vi "CALC_EQU_VAL.vi"(0 "VISA IN":refnum<visa-resource-name>, 5 "error in":errorcluster, 7 "Channel":i32) -> (14 "VISA Out":refnum<visa-resource-name>, 18 "EqValid?":bool, 19 "error out":errorcluster)   [LabVIEW 2018, in "PNA-X.lvlib"]
doc: "CALCulate<cnum>:EQUation:VALid? \n1504\n\n(Read-Write) Returns a boolean value to indicate if the current equation on the selected measurement \nfor the specified channel is valid. For equation processing to occur, the equation must be valid and \nON (CALC:EQU:STAT 1). \nSee Critical Note \nParameters \n<cnum> Channel number of the measurement. There must be a selected measurement \non that channel. If unspecified, <cnum> is set to 1. \nExamples CALC:EQU:VAL? \ncalculate2:equation:valid? \nReturn Type Boolean \n1 - equation is valid \n0 - equation is NOT valid \nDefault Not Applicable \n1505\n\nCalculate:Filter Commands \nControls the gating function used in time domain measurements. The gated range is specified with \neither (start / stop) or (center / span) commands. \nClick on a blue keyword to view the command details. \nSee Also \nExample Programs \nLearn about Gating \nSynchronizing the PNA and Controller \nSCPI Command Tree \nCritical Note: CALCulate commands act on the selected measurement. You can select one \nmeasurement for each channel using Calc:Par:Select"
uses:
  PNA-X.lvlib
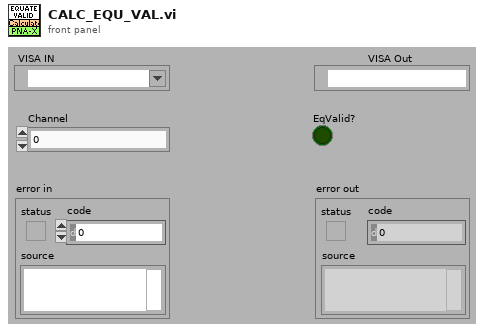
[diagram p1: front panel]
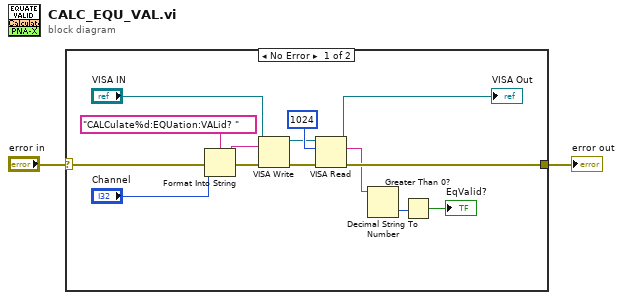
[diagram p0: block diagram]
diagram:
  n1 = case shown="No Error" "error in" {
    selector: "error in" -> [w16 w17]
    tunnel: [w8 w17] -> w1
    frame No Error {
      n2 = Format Into String(format string="CALCulate%d:EQUation:VALid? " ("Cmdline"), error in=w16, "Channel") -> (resulting string=w14:string, error out=w15:errorcluster)  [unwired: 1 in]
      n3 = VISA Write(VISA resource name="VISA IN", write buffer=w14, error in (no error)=w15) -> (VISA resource name out=w9:refnum<visa-resource-name>, error out=w11:errorcluster)  [unwired: 1 out]
      n4 = VISA Read(VISA resource name=w9, byte count=1024, error in (no error)=w11) -> (VISA resource name out=→"VISA Out":refnum<visa-resource-name>, read buffer=w5:string, error out=w8:errorcluster)  [unwired: 1 out]
      n5 = Decimal String To Number(string=w5) -> (number=w4:i32)  [unwired: 2 in, 1 out]
      n6 = Greater Than 0?(x=w4) -> (x > 0?=→"EqValid?":bool)
    }
    frame Error {
    }
  }
  "error out" <- w1
